vi "Get Routine.vi"(8 "error in (no error)":errorcluster, 11 "Item Ref in":T1 format="%.0x") -> (0 "error out":errorcluster, 2 "Routine":T2 {"Stop Parameters"."Response"."Byte Order" items=["Little Endian", "Big Endian"]; "Stop Parameters"."Response"."Data Type" items=["Signed", "Unsigned", "IEEE Float"]; "Stop Parameters"."Cmd"."Byte Order" items=["Little Endian", "Big Endian"]; "Stop Parameters"."Cmd"."Data Type" items=["Signed", "Unsigned", "IEEE Float"]; "Request Parameters"."Response"."Byte Order" items=["Little Endian", "Big Endian"]; "Request Parameters"."Response"."Data Type" items=["Signed", "Unsigned", "IEEE Float"]; "Request Parameters"."Cmd"."Byte Order" items=["Little Endian", "Big Endian"]; "Request Parameters"."Cmd"."Data Type" items=["Signed", "Unsigned", "IEEE Float"]; "Start Parameters"."Response"."Byte Order" items=["Little Endian", "Big Endian"]; "Start Parameters"."Response"."Data Type" items=["Signed", "Unsigned", "IEEE Float"]; "Start Parameters"."Cmd"."Byte Order" items=["Little Endian", "Big Endian"]; "Start Parameters"."Cmd"."Data Type" items=["Signed", "Unsigned", "IEEE Float"]}, 3 "Section Ref out":T1 format="%.0x")   [LabVIEW 2015, in "Diagnostics Addon System Explorer.lvlib"]
uses:
  Diagnostics Addon System Explorer.lvlib
  <vilib>/NI Veristand/Custom Device API/Custom Device Item Ref.ctl
  Shared/Types/Routine Paramaters.ctl
  Shared/Types/Command Response Signals.ctl
  Shared/Types/Signal Parameters.ctl
  Types/FG Action.ctl
  Get Signals.vi
  Type FG.vi
  Signal Parameters FG.vi
  <vilib>/NI Veristand/Custom Device API/NI VeriStand - Get Item Property.vi
  <vilib>/NI Veristand/Custom Device API/Get Item Property (U32).vi
  <vilib>/NI Veristand/Custom Device API/NI VeriStand - Set Item Property.vi
  <vilib>/NI Veristand/Custom Device API/Set Item Property (U32).vi
  Shared/SubVIs/GUID Lookup.vi
  <vilib>/NI Veristand/Custom Device API/NI VeriStand - Get Custom Device Channel Data.vi
  <vilib>/NI Veristand/Custom Device API/Get Item Property (String).vi
  <vilib>/NI Veristand/Custom Device API/Get Item Property (Double).vi
  <vilib>/NI Veristand/Custom Device API/Set Item Property (String).vi
  <vilib>/NI Veristand/Custom Device API/Set Item Property (Double).vi
  <vilib>/NI Veristand/Custom Device API/NI VeriStand - Get Item Children.vi
  <vilib>/NI Veristand/Custom Device Tools/Custom Device Utility Library/NI VeriStand - Search for Item by GUID.vi
  Shared/Diagnostics Addon Shared.lvlib
  <vilib>/NI Veristand/Custom Device API/Custom Device API.lvlib
  <vilib>/NI Veristand/Custom Device Tools/Custom Device Utility Library/Custom Device Utility Library.lvlib
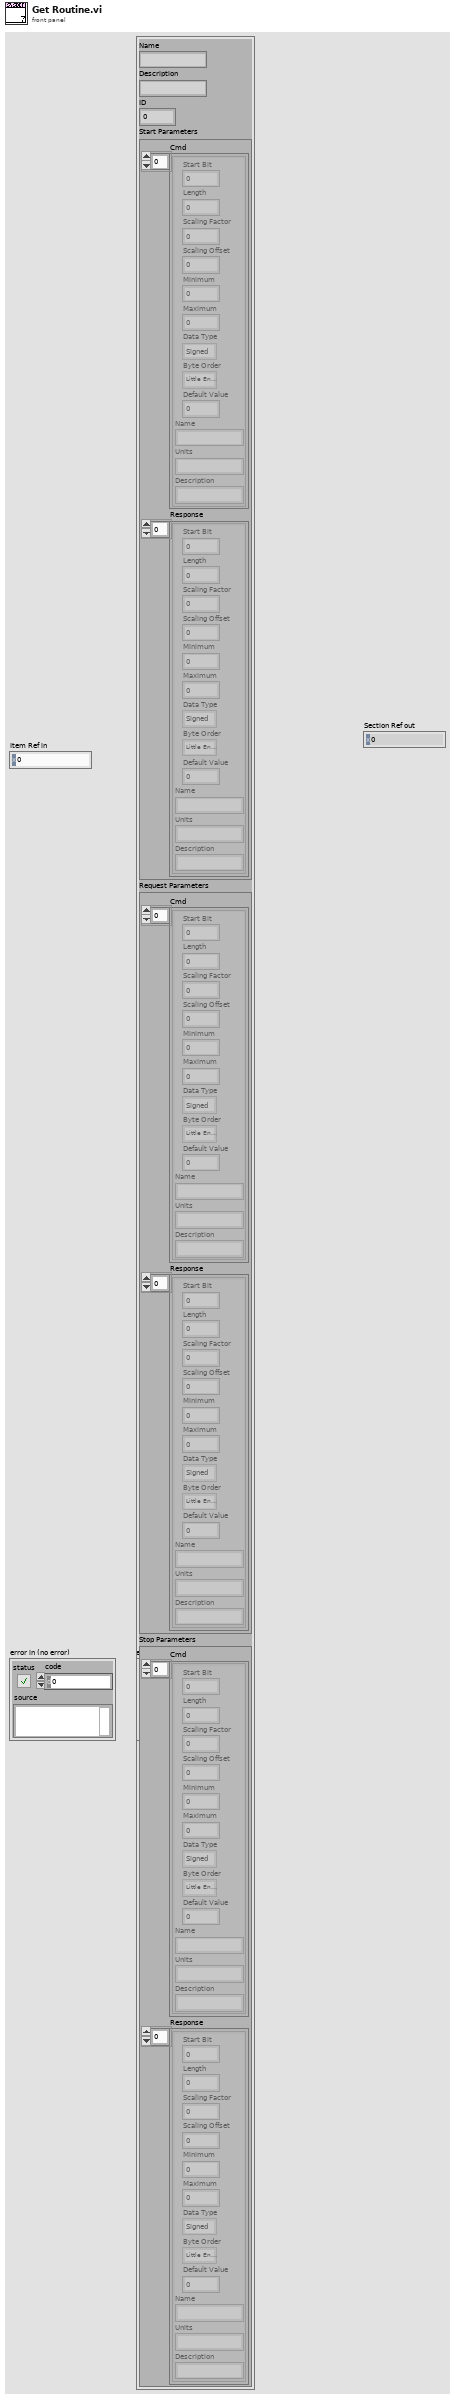
[diagram p1: front panel]
types:
  T1 = typedef "Custom Device API.lvlib/Custom Device Item Ref.ctl" = u64
  T2 = typedef "Diagnostics Addon Shared.lvlib/Routine Paramaters.ctl" = cluster{"Name":string, "Description":string, "ID":u16, "Start Parameters":T3, "Request Parameters":T3, "Stop Parameters":T3}
  T3 = typedef "Diagnostics Addon Shared.lvlib/Command Response Signals.ctl" = cluster{"Cmd":T4[], "Response":T4[]}
  T4 = typedef "Diagnostics Addon Shared.lvlib/Signal Parameters.ctl" = cluster{"Start Bit":u8, "Length":u8, "Scaling Factor":dbl, "Scaling Offset":dbl, "Minimum":dbl, "Maximum":dbl, "Data Type":u32, "Byte Order":u32, "Default Value":dbl, "Name":string, "Units":string, "Description":string}
  T5 = typedef "Diagnostics Addon System Explorer.lvlib/FG Action.ctl" = enum16{"Get", "Set"}
  T6 = typedef "Custom Device API.lvlib/Custom Device Item Info.ctl" = cluster{"Name":string, "Is Channel":bool, "GUID":string, "Is Waveform":bool}
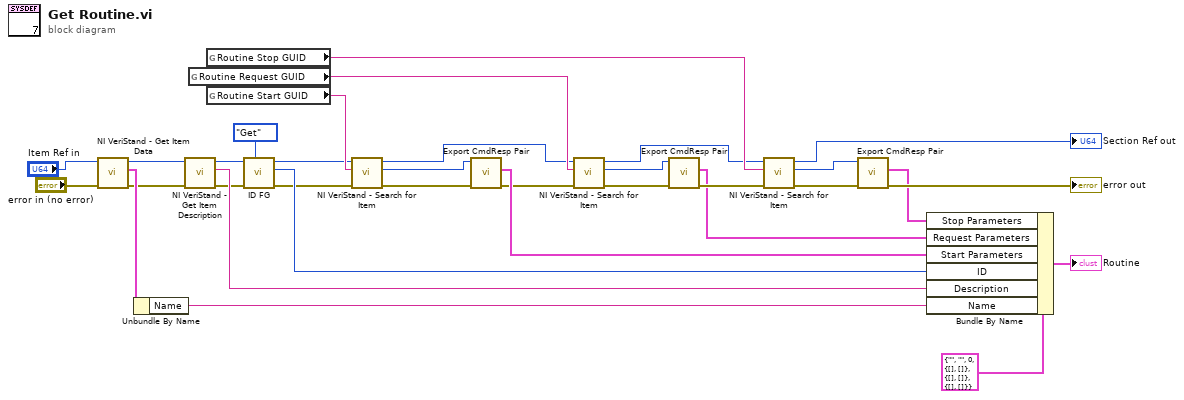
[diagram p0: block diagram]
diagram:
  n1 = call <vilib>:"NI VeriStand - Get Item Data.vi"("error in (no error)"="error in (no error)", "Item Ref in"="Item Ref in") -> ("error out"=w31:errorcluster, "Item Info"=w32:T6, "Item Ref out"=w29:T1)  [unwired: 6 in, 1 out]
  n2 = Unbundle By Name(w32) -> ("Name"=w33:string)
  n3 = call <vilib>:"NI VeriStand - Get Item Description.vi"("error in (no error)"=w31, "Item Ref in"=w29) -> ("error out"=w24:errorcluster, "Description"=w26:string, "Item Ref out"=w25:T1)  [unwired: 6 in, 1 out]
  n4 = global read "GUID Lookup.vi" "Routine Request GUID"() -> (w11:string)
  n5 = global read "GUID Lookup.vi" "Routine Stop GUID"() -> (w10:string)
  n6 = global read "GUID Lookup.vi" "Routine Start GUID"() -> (w12:string)
  n7 = call "ID FG.vi"("Action"=FG_Action."Get", "error in (no error)"=w24, "Device Item Ref in"=w25) -> ("error out"=w22:errorcluster, "ID"=w27:u32, "Device Item Ref out"=w7:T1)  [unwired: 6 in]
  n8 = call-poly <vilib>:"NI VeriStand - Search for Item.vi"("error in"=w22, "Item GUID"=w12, "Section Ref in"=w7) -> ("error out"=w15:errorcluster, "Item Ref"=w5:T1, "Section Ref out"=w6:T1)  [unwired: 5 in, 1 out]
  n9 = call "Export CmdResp Pair.vi"("error in (no error)"=w15, "Device Item Ref in"=w5) -> ("error out"=w18:errorcluster, "Signals"=w20:T3)  [unwired: 7 in, 1 out]
  n10 = call-poly <vilib>:"NI VeriStand - Search for Item.vi"("error in"=w18, "Item GUID"=w11, "Section Ref in"=w6) -> ("error out"=w14:errorcluster, "Item Ref"=w8:T1, "Section Ref out"=w9:T1)  [unwired: 5 in, 1 out]
  n11 = call "Export CmdResp Pair.vi"("error in (no error)"=w14, "Device Item Ref in"=w8) -> ("error out"=w17:errorcluster, "Signals"=w2:T3)  [unwired: 7 in, 1 out]
  n12 = call-poly <vilib>:"NI VeriStand - Search for Item.vi"("error in"=w17, "Item GUID"=w10, "Section Ref in"=w9) -> ("error out"=w13:errorcluster, "Item Ref"=w4:T1, "Section Ref out"=→"Section Ref out":T1)  [unwired: 5 in, 1 out]
  n13 = call "Export CmdResp Pair.vi"("error in (no error)"=w13, "Device Item Ref in"=w4) -> ("error out"=→"error out":errorcluster, "Signals"=w1:T3)  [unwired: 7 in, 1 out]
  n14 = Bundle By Name(cluster=T2 {"Name"="", "Description"="", "ID"=0, "Start Parameters"={"Cmd"=[], "Response"=[]}, "Request Parameters"={"Cmd"=[], "Response"=[]}, "Stop Parameters"={"Cmd"=[], "Response"=[]}} ("Routine"), "Stop Parameters"=w1, "Request Parameters"=w2, "Start Parameters"=w20, "ID"=w27, "Description"=w26, "Name"=w33) -> (→"Routine":T2)
